vi "Write Data Under SpecifiedCell.vi"(7 "name":string, 8 "error in":errorcluster caption="错误输入（无错误）", 9 "text":string caption="文本", 10 "Row count in":i32, 11 "report in":refnum<class "NI_report.lvclass"> caption="报表输入") -> (0 "error out":errorcluster caption="错误输出", 2 "Row count out":i32, 3 "report out":refnum<class "NI_report.lvclass"> caption="报表输出")   [LabVIEW 2016]
uses:
  <vilib>/Utility/NIReport.llb/NI_report.lvclass
  <vilib>/Utility/NIReport.llb/Append Report Text (str wrap).vi
  <vilib>/addons/_office/NI_ReportGenerationToolkit.lvlib
  <vilib>/Utility/NIReport.llb/Excel/NI_Excel.lvclass
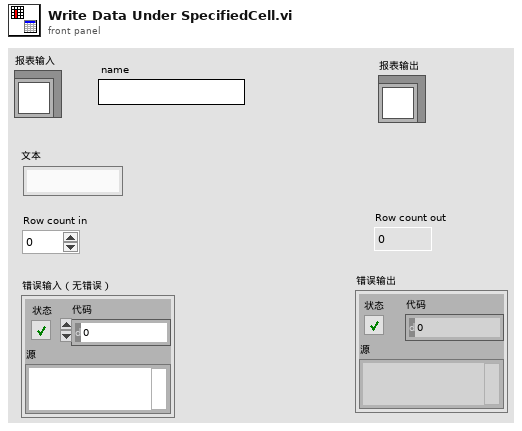
[diagram p1: front panel]
types:
  T1 = cluster{"position (excel)":cluster{"row":i32, "column":i32}, "name (excel)":string, "bookmark (word)":string}
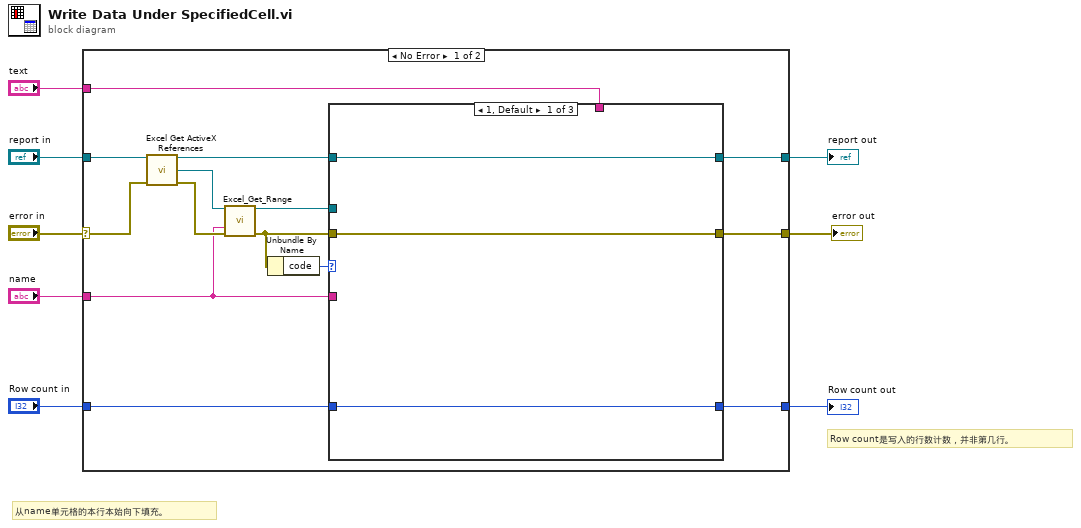
[diagram p0: block diagram]
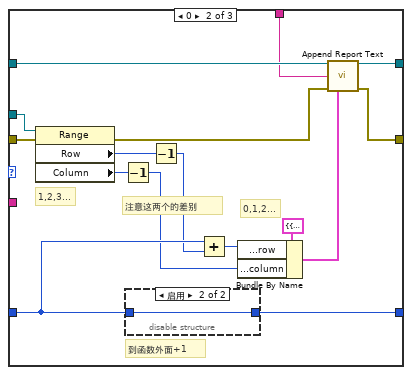
[diagram p2: hidden frame]
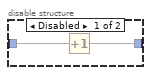
[diagram p3: hidden frame]
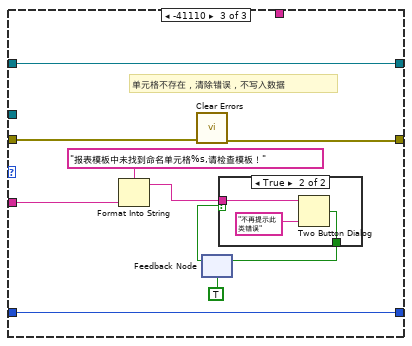
[diagram p4: hidden frame]
diagram:
  # "从name单元格的本行本始向下填充。"
  # "Row count是写入的行数计数，并非第几行。"
  n1 = case shown="No Error" "error in" {
    selector: "error in" -> [w14 w61]
    tunnel: "report in" -> [w21 w59]
    tunnel: "Row count in" -> [w12 w60]
    tunnel: [w17 w59] -> w6
    tunnel: [w13 w60] -> w5
    tunnel: "text" -> [w16 _]
    tunnel: [w15 w61] -> w3
    tunnel: "name" -> [w9 _]
    frame No Error {
      n2 = call <vilib>:"Excel Get ActiveX References.vi"("report in"=w21, "error in (no error)"=w14) -> ("report out"=w18:refnum<class "NI_report.lvclass">, "Excel._Worksheet"=w22:refnum<k7>, "error out"=w20:errorcluster)  [unwired: 7 in, 4 out]
      n3 = call <vilib>:"Excel_Get_Range.vi"("Excel._Worksheet"=w22, "name"=w9, "error in (no error)"=w20) -> ("Range"=w19:refnum<k7>, "error out"=w11:errorcluster)  [unwired: 2 in, 9 out]
      n4 = Unbundle By Name(w11) -> ("code"=w10:i32)
      n5 = case shown="1, Default" w10 {
        tunnel: w19 -> [_ w41 _]
        tunnel: w11 -> [w24 w26 w53]
        tunnel: w18 -> [w25 w37 w54]
        tunnel: [w25 w35 w54] -> w17
        tunnel: w16 -> [_ w33 _]
        tunnel: [w24 w32 w52] -> w15
        tunnel: [w23 w31 w51] -> w13
        tunnel: w12 -> [w23 w30 w51]
        tunnel: w9 -> [_ _ w50]
        frame 1, Default {
        }
        frame 0 {
          # "注意这两个的差别"
          # "0,1,2..."
          # "1,2,3..."
          # "到函数外面+1"
          n6 = property class="Range"(reference=w41, error in=w26) -> (error out=w36:errorcluster, "Row"=w28:i32, "Column"=w38:i32)  [unwired: 1 out]
          n7 = Decrement(x=w38) -> (x-1=w29:i32)
          n8 = disable-structure shown="启用" {
            disable-tunnel: w30 -> [w43 w44]
            disable-tunnel: [w42 w44] -> w31
            frame Disabled {
              n9 = Increment(x=w43) -> (x+1=w42:i32)
            }
            frame Enabled {
            }
          }
          n10 = Decrement(x=w28) -> (x-1=w27:i32)
          n11 = Add(x=w30, y=w27) -> (x+y=w39:i32)
          n12 = Bundle By Name(cluster=T1 {"position (excel)"={"row"=0, "column"=0}, "name (excel)"="", "bookmark (word)"=""} ("MS Office parameters"), "position (excel).row"=w39, "position (excel).column"=w29) -> (w34:T1)
          n13 = call-poly <vilib>:"Append Report Text.vi"("report in"=w37, "MS Office parameters"=w34, "text"=w33, "error in (no error)"=w36) -> ("report out"=w35:refnum<class "NI_report.lvclass">, "error out"=w32:errorcluster)  [unwired: 8 in, 2 out]
        }
        frame -41110 {
          # "单元格不存在，清除错误，不写入数据"
          n14 = Format Into String(format string="报表模板中未找到命名单元格%s,请检查模板！" ("格式字符串"), w50) -> (resulting string=w49:string)  [unwired: 2 in, 1 out]
          n15 = call <vilib>:"Clear Errors.vi"("error in (no error)"=w53) -> ("error out"=w52:errorcluster)  [unwired: 5 in, 1 out]
          n16 = feedback #1(TRUE) -> (w45:bool)
          n17 = case shown="True" w45 {
            selector: w45 -> [w55 _]
            tunnel: w49 -> [_ w57]
            tunnel: [w55 w56] -> w46
            frame False {
            }
            frame True {
              n18 = Two Button Dialog(message=w57, 1:"不再提示此类错误" ("F按钮名称（“取消”）")) -> (T button?=w56:bool)  [unwired: 1 in]
            }
          }
          n19 = feedback-in #1(w46) -> ()
        }
      }
    }
    frame Error {
    }
  }
  "report out" <- w6
  "error out" <- w3
  "Row count out" <- w5
